vi "Wait for Trigger.vi"(8 "error in (no error)":errorcluster, 11 "Pulse Controller in":refnum<class "Pulse Recorder.lvclass">) -> (0 "error out":errorcluster, 3 "Pulse Controller out":refnum<class "Pulse Recorder.lvclass">)   [LabVIEW 2015, in "Pulse Recorder.lvclass"]
uses:
  Pulse Recorder.lvclass
  <vilib>/ActorFramework/Actor/Actor.lvclass/Actor.ctl
  <vilib>/ActorFramework/Message Enqueuer/Message Enqueuer.lvclass/Message Enqueuer.ctl
  Pulse Recorder.lvclass/Pulse Recorder.ctl
  <vilib>/ActorFramework/Message Enqueuer/Init from Existing Queue.vi
  <vilib>/ActorFramework/Time-Delayed Send Message/Time-Delayed Send Message.vi
  <vilib>/ActorFramework/Message Enqueuer/Message Enqueuer.lvclass
  Pulse Controller Messages/Wait for Trigger Msg/Wait for Trigger Msg.lvclass
  <vilib>/ActorFramework/Actor/Actor.lvclass
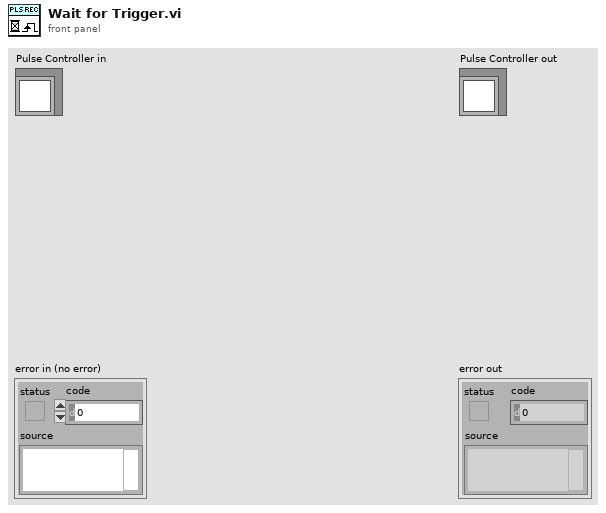
[diagram p1: front panel]
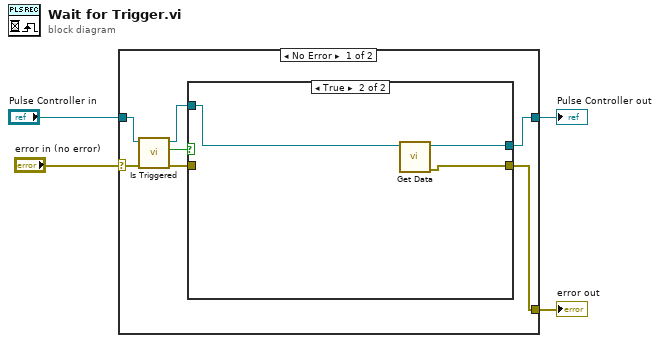
[diagram p0: block diagram]
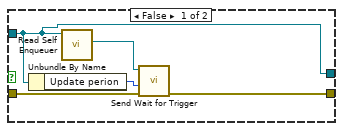
[diagram p2: hidden frame]
diagram:
  n1 = case shown="No Error" "error in (no error)" {
    selector: "error in (no error)" -> [w10 w21]
    tunnel: [w7 w21] -> w3
    tunnel: [w5 w20] -> w1
    tunnel: "Pulse Controller in" -> [w11 w20]
    frame No Error {
      n2 = call-dynamic "Is Triggered.vi"("error in (no error)"=w10, "Pulse Controller in"=w11) -> ("error out"=w8:errorcluster, "Triggered"=w9:bool, "Pulse Controller out"=w6:refnum<class "Pulse Recorder.lvclass">)  [unwired: 7 in]
      n3 = case shown="True" w9 {
        tunnel: w6 -> [w12 w19]
        tunnel: w8 -> [w14 _]
        tunnel: [w13 w17] -> w7
        tunnel: [w12 w18] -> w5
        frame False {
          n4 = Unbundle By Name(w12) -> ("Update perion"=w16:i32)
          n5 = call <vilib>:"Read Self Enqueuer.vi"("Actor"=w12) -> ("Self Enqueuer"=w15:refnum<class "Message Enqueuer.lvclass">)  [unwired: 10 in]
          n6 = call "Send Wait for Trigger.vi"("error in (no error)"=w14, "Milliseconds To Wait"=w16, "Message Enqueuer"=w15) -> ("error out"=w13:errorcluster)  [unwired: 6 in, 2 out]
        }
        frame True {
          n7 = call-dynamic "Get Data.vi"("Pulse Recorder in"=w19) -> ("error out"=w17:errorcluster, "Pulse Recorder out"=w18:refnum<class "Pulse Recorder.lvclass">)  [unwired: 9 in]
        }
      }
    }
    frame Error {
    }
  }
  "error out" <- w3
  "Pulse Controller out" <- w1
